vi "phase difference testing.vi"() -> ()   [LabVIEW 2017]
panel:
  in  "stop (F)":bool
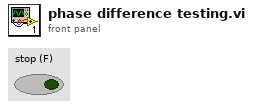
[diagram p1: front panel]
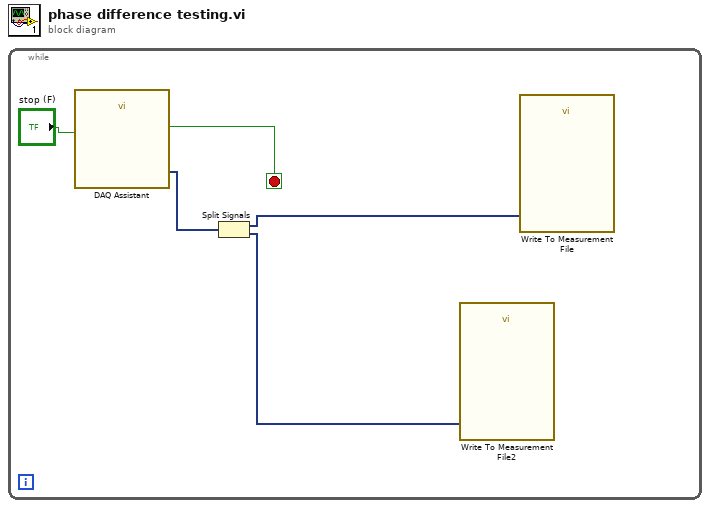
[diagram p0: block diagram]
diagram:
  n1 = while {
    stop <- w4 stop-if-true
    n2 = call "DAQ Assistant"("stop (F)"="stop (F)") -> ("data"=w3:dynamicdata, "stopped"=w4:bool)  [unwired: 15 in, 2 out]
    n3 = Split Signals(w3) -> (w2:dynamicdata, w1:dynamicdata)  [unwired: 2 in]
    n4 = call "Write To Measurement File2"("Signals"=w1) -> ()  [unwired: 16 in, 3 out]
    n5 = call "Write To Measurement File"("Signals"=w2) -> ()  [unwired: 16 in, 3 out]
  }
